vi "Write TID.vi"(8 "error in (no error)":errorcluster, 10 "TID":u8, 11 "23-Equipment Sends Information to Host in":refnum<class "23-Equipment Sends Information to Host.lvclass">) -> (0 "error out":errorcluster, 3 "23-Equipment Sends Information to Host out":refnum<class "23-Equipment Sends Information to Host.lvclass">)   [LabVIEW 2020, in "SECS Scenarios.lvlib" / "23-Equipment Sends Information to Host.lvclass"]
uses:
  23-Equipment Sends Information to Host.lvclass
  23-Equipment Sends Information to Host.lvclass/23-Equipment Sends Information to Host.ctl
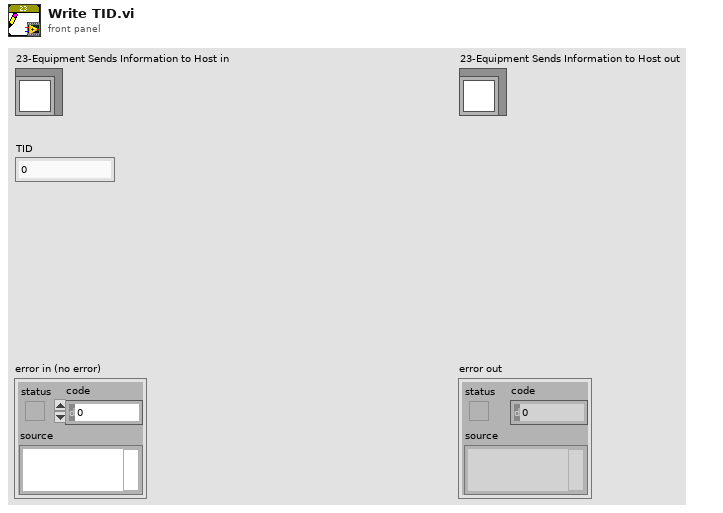
[diagram p1: front panel]
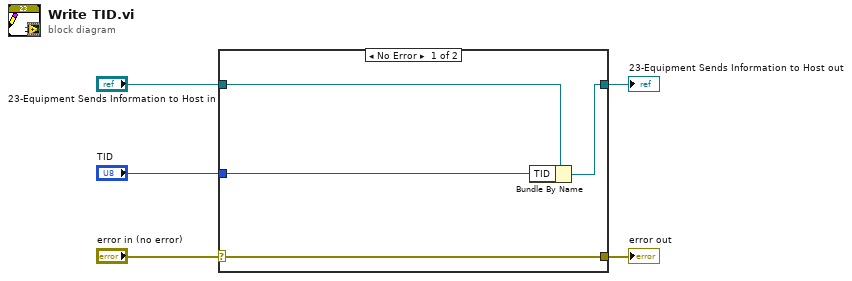
[diagram p0: block diagram]
diagram:
  n1 = case shown="No Error" "error in (no error)" {
    selector: "error in (no error)" -> [w9 w10]
    tunnel: [w9 w10] -> w4
    tunnel: [w7 w11] -> w2
    tunnel: "23-Equipment Sends Information to Host in" -> [w8 w11]
    tunnel: "TID" -> [w6 _]
    frame No Error {
      n2 = Bundle By Name(cluster=w8, "TID"=w6) -> (w7:refnum<class "23-Equipment Sends Information to Host.lvclass">)
    }
    frame Error {
    }
  }
  "error out" <- w4
  "23-Equipment Sends Information to Host out" <- w2
